vi "Framework.Rx.End.vi"(8 "error in (no error)":errorcluster, 11 "Framework in":refnum<class "Framework.lvclass">) -> (0 "error out":errorcluster, 3 "Framework out":refnum<class "Framework.lvclass">)   [LabVIEW 2017, in "DSF Core.lvlib" / "Framework.lvclass"]
uses:
  Framework.lvclass
  Framework.lvclass/Framework.ctl
  Status/Framework Status.lvclass/Framework Status.ctl
  Status/Framework Performance.lvclass/Framework Performance.ctl
  <vilib>/NI/Memory Manager/Classes/Pointer/Memory.Pointer.lvclass/Memory.Pointer.ctl
  <vilib>/NI/Memory Manager/Classes/Pointer/Memory.Pointer.Write.vi
  <vilib>/NI/Memory Manager/Classes/Pointer/Memory.Pointer.Write.0D.U32.vi
  <vilib>/NI/Memory Manager/Classes/Pointer/Memory.Pointer.Write.No Check.0D.U32.vi
  <vilib>/NI/Memory Manager/Classes/Pointer/Memory.Pointer.Parameter Check.Null Pointer.vi
  <vilib>/NI/Memory Manager/Classes/Pointer/Memory.Pointer.Parameter Check.Subset.vi
  <vilib>/NI/Memory Manager/Classes/Pointer/Memory.Pointer.Get Address.vi
  <vilib>/NI/Memory Manager/Classes/Pointer/Memory.Pointer.Errors.vi
  <vilib>/NI/Memory Manager/Classes/Pointer/Memory.Pointer.Errors.Null Pointer.vi
  <vilib>/NI/Memory Manager/Classes/Pointer/Memory.Pointer.Errors.Out of Bounds.vi
  <vilib>/NI/Memory Manager/Classes/Pointer/Memory.Pointer.Get Size.vi
  <vilib>/NI/Memory Manager/Classes/Pointer/Memory.Pointer.Errors.Create Error.vi
  <vilib>/NI/Memory Manager/VIs/Source.Write.String.vi
  <vilib>/NI/Memory Manager/Classes/Pointer/Memory.Pointer.Errors.Write Pointer Size.vi
  <vilib>/NI/Memory Manager/VIs/Source.Write.Scalar.Base10.vi
  <vilib>/NI/Memory Manager/VIs/Source.Write.Scalar.Base10 (U64).vi
  <vilib>/NI/Memory Manager/VIs/New Error Cluster Constant.vi
  <vilib>/NI/Memory Manager/VIs/New Error Cluster Constant (512B).vi
  <vilib>/NI/Memory Manager/VIs/Error Cluster.Set Status.vi
  <vilib>/NI/Memory Manager/VIs/Error Cluster.Set Code.vi
  <vilib>/NI/Memory Manager/VIs/Error Cluster.Set VI Source.vi
  <vilib>/NI/Memory Manager/Constants/Memory.Constants.vi
  <vilib>/NI/Memory Manager/Constants/Memory.Constants.Library Name.vi
  <vilib>/NI/Memory Manager/Classes/Pointer/Memory.Pointer.Errors.Get Info.vi
  Status/Framework Status.lvclass
  Status/Framework Performance.lvclass
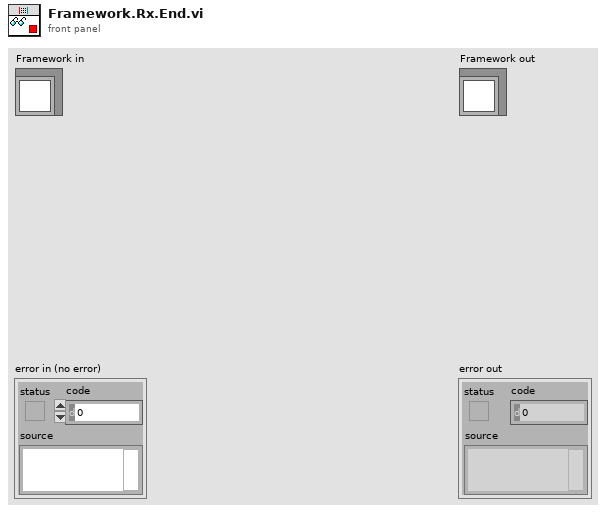
[diagram p1: front panel]
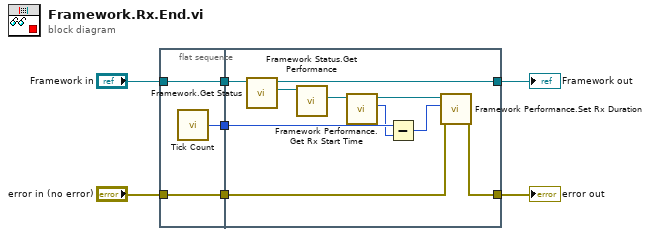
[diagram p0: block diagram]
diagram:
  n1 = flat-sequence {
    tunnel: "Framework in" -> [w10]
    tunnel: [w10] -> w5
    tunnel: [w9] -> w4
    tunnel: "error in (no error)" -> [w8]
    tunnel: [w8] -> w2
    tunnel: [w18] -> w6
    tunnel: w5 -> [w19]
    tunnel: w4 -> [w16]
    tunnel: w2 -> [w12]
    tunnel: [w11] -> w1
    frame #0 {
      n2 = call "Tick Count"() -> ("Tick Count(uSec)"=w9:u32)
    }
    frame #1 {
      n3 = call "Framework.Get Status.vi"("Framework in"=w19) -> ("Status"=w20:refnum<class "Framework Status.lvclass">, "Framework out"=w18:refnum<class "Framework.lvclass">)  [unwired: 9 in]
      n4 = call "Framework Status.Get Performance.vi"("Framework Status in"=w20) -> ("Framework Performance"=w17:refnum<class "Framework Performance.lvclass">)  [unwired: 9 in, 1 out]
      n5 = call "Framework Performance.Get Rx Start Time.vi"("Framework Performance in"=w17) -> ("Rx start time"=w15:u32, "Framework Performance out"=w14:refnum<class "Framework Performance.lvclass">)  [unwired: 9 in]
      n6 = Subtract(x=w16, y=w15) -> (x-y=w13:u32)
      n7 = call "Framework Performance.Set Rx Duration.vi"("error in (no error)"=w12, "rx duration"=w13, "Framework Performance in"=w14) -> ("error out"=w11:errorcluster)  [unwired: 7 in, 1 out]
    }
  }
  "error out" <- w1
  "Framework out" <- w6
